vi "InstantiateNewShoot.vi"(8 "error in":errorcluster, 11 "ShootsRef in":T1[](array[typedef])) -> (0 "error out":errorcluster, 3 "ShootsRef out":T1[](array[typedef]))   [LabVIEW 2017]
uses:
  ManRef_ShootData.ctl
  Spaceship/Spaceship_mods.ctl
  Spaceship/Spaceship_data.ctl
  GameConfig/GameConfig_data.ctl
  Spaceship/Shoot/Shoot_data.ctl
  Spaceship/Shoot/Shoot_states.ctl
  HoldData/DataForColision.ctl
  HoldData/HoldData_mods.ctl
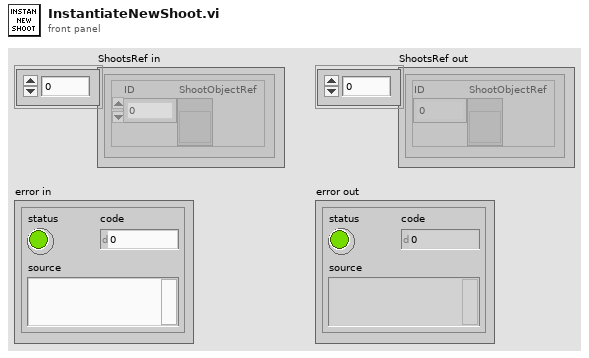
[diagram p1: front panel]
types:
  T1 = typedef "ManRef_ShootData.ctl" = cluster{"ID":i32, "ShootObjectRef":refnum<vi>}
  T2 = typedef "GameConfig_data.ctl" = cluster{"SpaceShip":cluster{"Angle":dbl, "SideLenght":dbl, "MaxLinearVeloc":dbl, "MaxAngularVeloc":dbl, "LinearAceleration":dbl, "AngularAceleration":dbl}, "Physics":cluster{"LinearDragFactor":dbl, "AngularDragFactor":dbl}, "Asteroids":cluster{"MaxSize":dbl, "MaxDivisions":i32, "MaxVeloc":dbl, "MinVeloc":dbl, "Fill":bool}, "Environment":cluster{"MaxAsteroids":i32, "TimeIncrement":dbl, "AsterProbCreation":dbl, "LogEnabled":bool}, "Shots":cluster{"MinTimeShots":dbl, "ShotSize":dbl, "ShotSpeed":dbl}}
  T3 = typedef "HoldData_mods.ctl" = enum16{"Init", "NewAster", "UpdateAster", "RemoveAster", "GetAsterData", "NewShoot", "UpdateShoot", "RemoveShoot", "GetShootData", "End"}
  T4 = typedef "DataForColision.ctl" = cluster{"X":dbl, "Y":dbl, "Size":dbl, "ID":i32}
  T5 = typedef "Shoot_states.ctl" = enum16{"Init", "Move", "Draw", "Destroy"}
  T6 = typedef "Shoot_data.ctl" = cluster{"Direction":dbl, "displayRef":refnum<vi>, "Max X":dbl, "Max Y":dbl, "Xpos":dbl, "Ypos":dbl, "ID":i32, "Config":T2}
  T7 = typedef "Spaceship_data.ctl" = cluster{"Angle":dbl, "XVeloc":dbl, "YVeloc":dbl, "AngVeloc":dbl, "GameConfig_data":T2, "Xpos":dbl, "Ypos":dbl, "Xmax":dbl, "Ymax":dbl}
  T8 = typedef "Spaceship_mods.ctl" = enum16{"Init", "Move", "Rotate", "Translate", "GetData", "End"}
  T9 = typedef "LVBoundsTypeDef.ctl" = cluster{"Width":u32, "Height":u32}
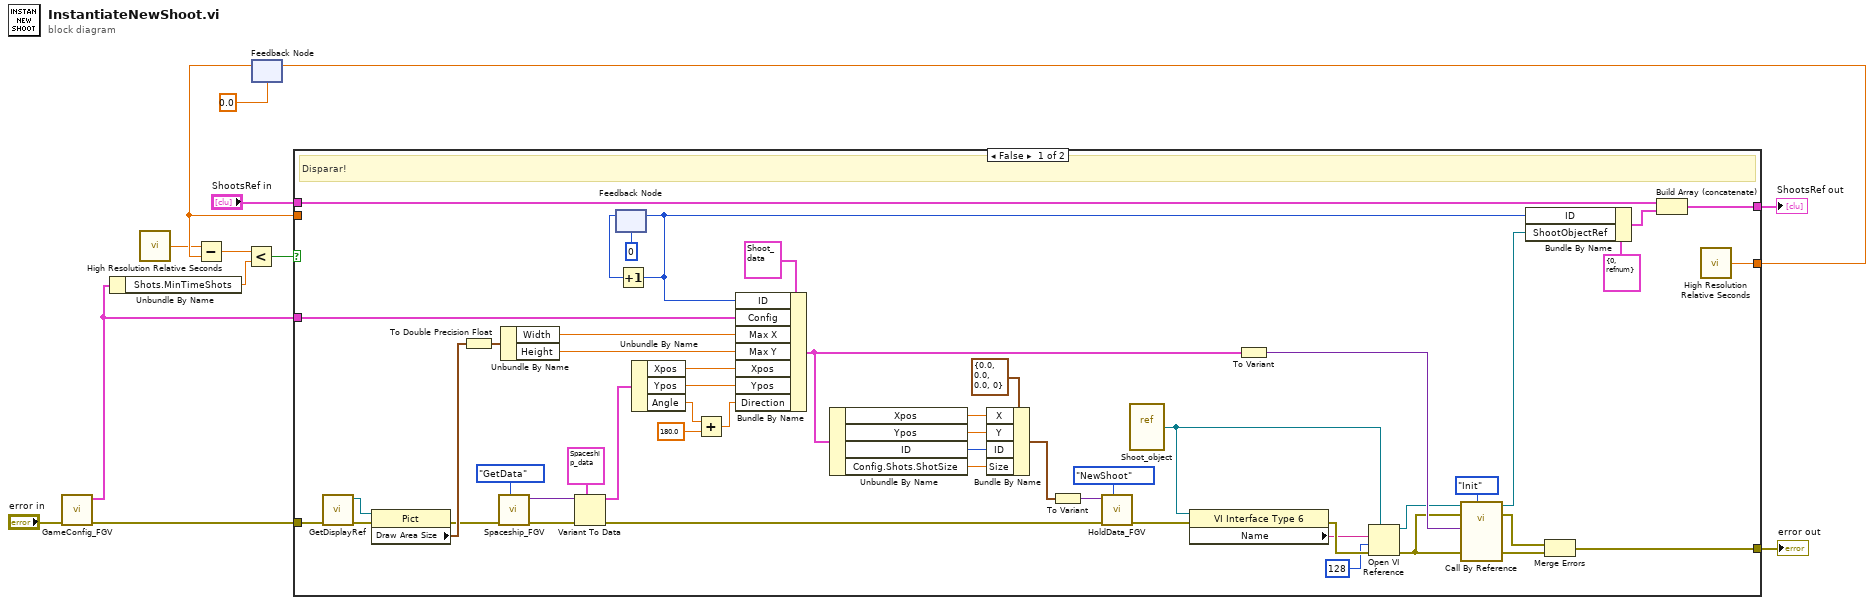
[diagram p0: block diagram]
diagram:
  n1 = call "GameConfig_FGV.vi"("error in"="error in") -> ("error out"=w9:errorcluster, "Config"=w1:T2)  [unwired: 9 in]
  n2 = Unbundle By Name(w1) -> ("Shots.MinTimeShots"=w5:dbl)
  n3 = call <vilib>:"High Resolution Relative Seconds.vi"() -> ("relative seconds"=w2:dbl)
  n4 = feedback #1(0.0 ("relative seconds")) -> (w8:dbl)
  n5 = Subtract(x=w2, y=w8) -> (x-y=w4:dbl)
  n6 = Less?(x=w4, y=w5) -> (x < y?=w6:bool)
  n7 = case shown="False" w6 {
    tunnel: [w64 w67] -> w7
    tunnel: w8 -> [_ w67]
    tunnel: w9 -> [w31 w65]
    tunnel: [w46 w65] -> w10
    tunnel: "ShootsRef in" -> [w39 w66]
    tunnel: [w38 w66] -> w12
    tunnel: w1 -> [w36 _]
    frame False {
      # "Disparar!"
      n8 = call "GetDisplayRef.vi"("error in"=w31) -> ("error out"=w35:errorcluster, "Picture out"=w34:refnum<vi>)  [unwired: 9 in]
      n9 = property class="Pict"(reference=w34, error in=w35) -> (error out=w30:errorcluster, "Draw Area Size"=w33:T9)  [unwired: 1 out]
      n10 = To Double Precision Float(number=w33) -> (double precision float=w32:cluster{"Width":dbl, "Height":dbl})
      n11 = call "Spaceship_FGV.vi"("Spaceship_mods"=Spaceship_mods."GetData", "error in"=w30) -> ("error out"=w62:errorcluster, "DataOut"=w37:variant)  [unwired: 8 in]
      n12 = Unbundle By Name(w32) -> ("Width"=w29:dbl, "Height"=w28:dbl)
      n13 = Variant To Data(error in=w62, type=T7 {"Angle"=0.0, "XVeloc"=0.0, "YVeloc"=0.0, "AngVeloc"=0.0, "GameConfig_data"={"SpaceShip"={"Angle"=30.0, "SideLenght"=2.0, "MaxLinearVeloc"=10.0, "MaxAngularVeloc"=10.0, "LinearAceleration"=1.0, "AngularAceleration"=1.0}, "Physics"={"LinearDragFactor"=1.0, "AngularDragFactor"=1.0}, "Asteroids"={"MaxSize"=6.0, "MaxDivisions"=3, "MaxVeloc"=8.0, "MinVeloc"=1.0, "Fill"=FALSE}, "Environment"={"MaxAsteroids"=10, "TimeIncrement"=0.1, "AsterProbCreation"=0.1, "LogEnabled"=FALSE}, "Shots"={"MinTimeShots"=10.0, "ShotSize"=0.1, "ShotSpeed"=0.1}}, "Xpos"=0.0, "Ypos"=0.0, "Xmax"=0.0, "Ymax"=0.0} ("Spaceship_data out"), Variant=w37) -> (data=w60:T7, error out=w18:errorcluster)
      n14 = feedback #2(0) -> (w52:i32)
      n15 = Increment(x=w52) -> (x+1=w59:i32)
      n16 = feedback-in #2(w59) -> ()
      n17 = Unbundle By Name(w60) -> ("Xpos"=w42:dbl, "Ypos"=w41:dbl, "Angle"=w16:dbl)
      n18 = Add(x=w16, y=180.0) -> (x+y=w15:dbl)
      n19 = Bundle By Name(cluster=T6 {"Direction"=0.0, "displayRef"=refnum, "Max X"=0.0, "Max Y"=0.0, "Xpos"=0.0, "Ypos"=0.0, "ID"=0, "Config"={"SpaceShip"={"Angle"=30.0, "SideLenght"=2.0, "MaxLinearVeloc"=10.0, "MaxAngularVeloc"=10.0, "LinearAceleration"=1.0, "AngularAceleration"=1.0}, "Physics"={"LinearDragFactor"=1.0, "AngularDragFactor"=1.0}, "Asteroids"={"MaxSize"=6.0, "MaxDivisions"=3, "MaxVeloc"=8.0, "MinVeloc"=1.0, "Fill"=FALSE}, "Environment"={"MaxAsteroids"=10, "TimeIncrement"=0.1, "AsterProbCreation"=0.1, "LogEnabled"=FALSE}, "Shots"={"MinTimeShots"=10.0, "ShotSize"=0.1, "ShotSpeed"=0.1}}} ("ShootData"), "ID"=w59, "Config"=w36, "Max X"=w29, "Max Y"=w28, "Xpos"=w42, "Ypos"=w41, "Direction"=w15) -> (w19:T6)
      n20 = Unbundle By Name(w19) -> ("Xpos"=w26:dbl, "Ypos"=w25:dbl, "ID"=w24:i32, "Config.Shots.ShotSize"=w20:dbl)
      n21 = Bundle By Name(cluster=T4 {"X"=0.0, "Y"=0.0, "Size"=0.0, "ID"=0} ("DataForColision"), "X"=w26, "Y"=w25, "ID"=w24, "Size"=w20) -> (w23:T4)
      n22 = To Variant(anything=w23) -> (Variant=w22:variant)
      n23 = call "HoldData_FGV.vi"("HoldData_mods"=HoldData_mods."NewShoot", "error in"=w18, "DataIn"=w22) -> ("error out"=w17:errorcluster)  [unwired: 7 in, 1 out]
      n24 = vi-ref "Shoot_object.vi"() -> (w51:refnum<vi>)
      n25 = property class="VI Interface Type 6"(reference=w51, error in=w17) -> (error out=w54:errorcluster, "Name"=w50:string)  [unwired: 1 out]
      n26 = To Variant(anything=w19) -> (Variant=w58:variant)
      n27 = Open VI Reference(type specifier VI Refnum (for type only)=w51, vi path=w50, options=128, error in (no error)=w54) -> (vi reference=w53:refnum<vi>, error out=w55:errorcluster)  [unwired: 2 in]
      n28 = call-by-ref "?"(reference=w53, error in=w55, "Shoot_states"=Shoot_states."Init", "error in"=w55, "DataIn"=w58) -> (reference out=w44:refnum<vi>, error out=w57:errorcluster, 0:"error out"=w56:errorcluster)  [unwired: 8 in]
      n29 = Bundle By Name(cluster=T1 {"ID"=0, "ShootObjectRef"=refnum} ("ShootData"), "ID"=w59, "ShootObjectRef"=w44) -> (w40:T1)
      n30 = Merge Errors(w57, w56) -> (w46:errorcluster)
      n31 = Build Array (concatenate)(w39, w40) -> (w38:T1[])
      n32 = call <vilib>:"High Resolution Relative Seconds.vi"() -> ("relative seconds"=w64:dbl)
    }
    frame True {
      # "Não disparar"
    }
  }
  "ShootsRef out" <- w12
  "error out" <- w10
  n33 = feedback-in #1(w7) -> ()
